vi "Drive Motor Joysticks.vi"(8 "Boost?":bool, 9 "Turn":dbl, 10 "Throttle":dbl) -> (2 "TEleop Drive command":T1)   [LabVIEW 2019]
uses:
  .Team Code/Robot Global Data.vi
  Drive Mode Typedef.ctl
  Drive Command Typedef.ctl
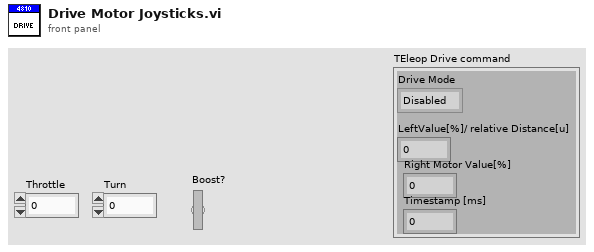
[diagram p1: front panel]
types:
  T1 = typedef "Drive Command Typedef.ctl" = cluster{"Drive Mode":T2, "LeftValue[%]/ relative Distance[u]":dbl, "Right Motor Value[%]":dbl, "Timestamp [ms]":dbl}
  T2 = typedef "Drive Mode Typedef.ctl" = enum16{"Disabled", "Auto-align", "Drive Distance", "Turn to angle", "Driver"}
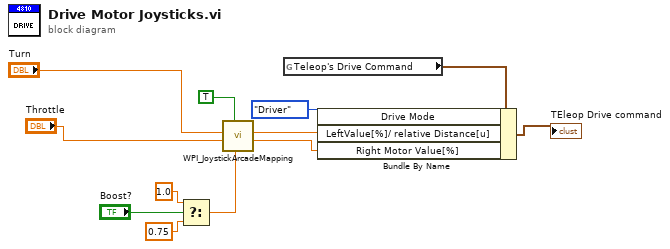
[diagram p0: block diagram]
diagram:
  n1 = Select(t=1.0, s="Boost?", f=0.75) -> (s? t:f=w5:dbl)
  n2 = call <vilib>:"WPI_JoystickArcadeMapping.vi"("Max Output"=w5, "Square Inputs"=TRUE, "Y axis value"="Throttle", "X axis value"="Turn") -> ("Right Motor Value"=w2:dbl, "Left Motor Value"=w3:dbl)  [unwired: 6 in]
  n3 = global read "Robot Global Data.vi" "Teleop's Drive Command"() -> (w9:T1)
  n4 = Bundle By Name(cluster=w9, "Drive Mode"=Drive_Mode_Typedef."Driver", "LeftValue[%]/ relative Distance[u]"=w3, "Right Motor Value[%]"=w2) -> (→"TEleop Drive command":T1)
